vi "LOERN_AdaptToInputs.vi"(0 "XRef":T9, 1 "Term Types":T6, 2 "State In":T1={"Inputs"=1, "SelectedIndex"=0, "ClassInfo"=[]}) -> (14 "Reply":T4, 15 "Fatal Error Out":T3, 16 "State Out":T1={"Inputs"=1, "SelectedIndex"=0, "ClassInfo"=[]})   [LabVIEW 2016, in "LV Object Event Registration Node.xnode"]
uses:
  LV Object Event Registration Node.xnode
  <vilib>/XNodeSupport/XNodeXNodeRef.ctl
  <vilib>/XNodeSupport/XNodeTermTypeIDPairs.ctl
  <vilib>/XNodeSupport/XNodeTermTypeIDPair.ctl
  <vilib>/XNodeSupport/XNodeType.ctl
  <vilib>/XNodeSupport/XNodeString.ctl
  LOERN_State.ctl
  LOERN_ClassInfo.ctl
  <vilib>/XNodeSupport/XNodeStringArray.ctl
  <vilib>/XNodeSupport/XNodeErrorCluster.ctl
  <vilib>/Utility/Data Type/NI_Data Type.lvlib
  <vilib>/XNodeSupport/NI_XNodeSupport.lvlib
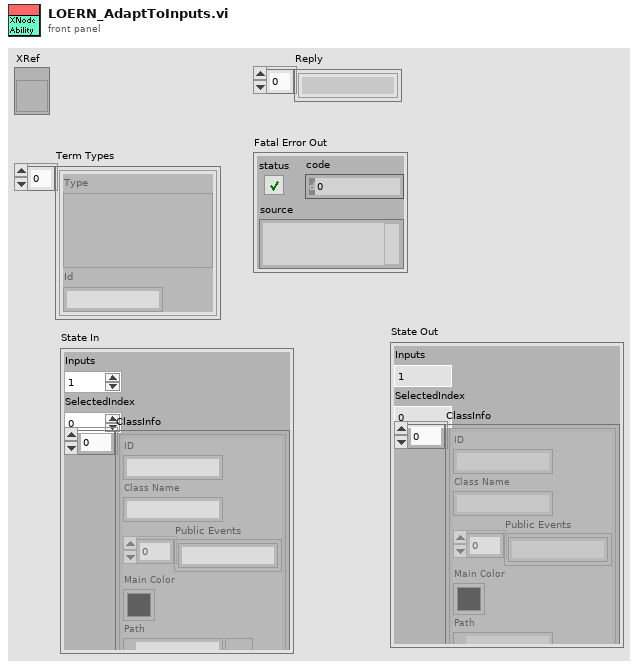
[diagram p1: front panel]
types:
  T1 = typedef "LV Object Event Registration Node.xnode/LOERN_State.ctl" = cluster{"Inputs":u16, "SelectedIndex":i16, "ClassInfo":T2[]}
  T2 = typedef "LV Object Event Registration Node.xnode/LOERN_ClassInfo.ctl" = cluster{"ID":string, "Class Name":string, "Public Events":string[], "Main Color":u32, "Path":path}
  T3 = typedef "NI_XNodeSupport.lvlib/XNodeErrorCluster.ctl" = errorcluster
  T4 = typedef "NI_XNodeSupport.lvlib/XNodeStringArray.ctl" = T5[]
  T5 = typedef "NI_XNodeSupport.lvlib/XNodeString.ctl" = string
  T6 = typedef "NI_XNodeSupport.lvlib/XNodeTermTypeIDPairs.ctl" = T7[]
  T7 = typedef "NI_XNodeSupport.lvlib/XNodeTermTypeIDPair.ctl" = cluster{"Type":T8, "Id":T5}
  T8 = typedef "NI_XNodeSupport.lvlib/XNodeType.ctl" = variant
  T9 = typedef "NI_XNodeSupport.lvlib/XNodeXNodeRef.ctl" = refnum<vi>
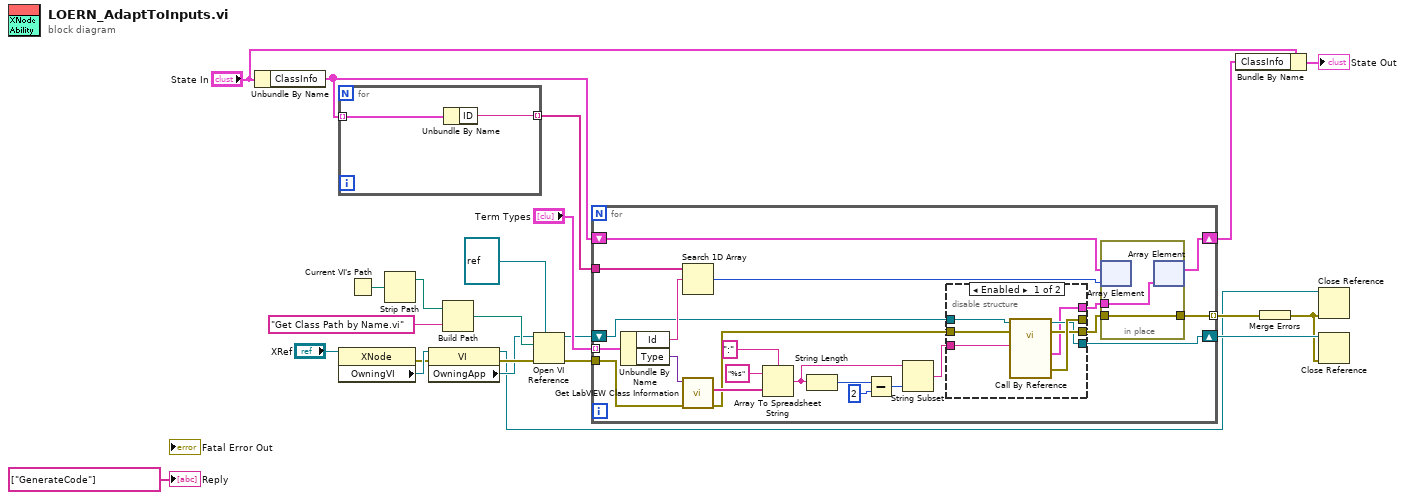
[diagram p0: block diagram]
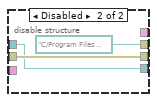
[diagram p2: hidden frame]
diagram:
  n1 = Unbundle By Name("State In") -> ("ClassInfo"=w21:T2[])
  n2 = for {
    tunnel: w21 -> [w25] mode=indexing
    tunnel: [w24] -> w22 mode=indexing
    n3 = Unbundle By Name(w25) -> ("ID"=w24:string)
  }
  n4 = property class="XNode"(reference="XRef") -> (error out=w12:errorcluster, "OwningVI"=w17:refnum<vi>)  [unwired: 1 in, 1 out]
  n5 = Current VI's Path() -> (path=w11:path)
  n6 = Strip Path(path=w11) -> (stripped path=w10:path)  [unwired: 1 out]
  n7 = property class="VI"(reference=w17, error in=w12) -> (reference out=w2:refnum<vi>, error out=w13:errorcluster, "OwningApp"=w7:refnum<vi>)
  n8 = Build Path(base path=w10, name or relative path="Get Class Path by Name.vi") -> (appended path=w8:path)
  n9 = Open VI Reference(type specifier VI Refnum (for type only)=refnum<vi> refnum, application reference (local)=w7, vi path=w8, error in (no error)=w13) -> (vi reference=w15:refnum<vi>, error out=w14:errorcluster)  [unwired: 2 in]
  n10 = for {
    tunnel: "Term Types" -> [w47] mode=indexing
    tunnel: w22 -> [w46]
    shift-right: [w42] -> w19
    shift-left: w21 -> [w44]
    tunnel: w14 -> [w29]
    shift-right: [w28] -> w5
    shift-left: w15 -> [w41]
    tunnel: [w27] -> w4 mode=indexing
    n11 = Unbundle By Name(w47) -> ("Id"=w45:T5, "Type"=w40:T8)
    n12 = Search 1D Array(1D array=w46, element=w45) -> (index of element=w43:i32)  [unwired: 1 in]
    n13 = call <vilib>:"Get LabVIEW Class Information.vi"("error in (no error)"=w29, "Variant"=w40) -> ("error out"=w30:errorcluster, "Qualified LabVIEW Class Name"=w37:string[])  [unwired: 7 in, 1 out]
    n14 = Array To Spreadsheet String(delimiter (Tab)=":", array=w37, 3:"%s" ("format string")) -> (spreadsheet string=w36:string)
    n15 = String Length(string=w36) -> (length=w35:i32)
    n16 = Subtract(x=w35, y=2) -> (x-y=w33:i32)
    n17 = String Subset(string=w36, length (rest)=w33) -> (substring=w32:string)  [unwired: 1 in]
    n18 = disable-structure shown="Enabled" {
      disable-tunnel: w41 -> [w54 w55]
      disable-tunnel: [w53 path "C:/Program Files (x86)/National Instruments/LabVIEW 2016/vi.lib/LIEF/Image Editor Handler/Image Editor Handler.lvclass"] -> _
      disable-tunnel: w32 -> [w52 _]
      disable-tunnel: [w51 w56] -> w31
      disable-tunnel: w30 -> [w50 w56]
      disable-tunnel: [w49 w55] -> w28
      disable-tunnel: [w48 _] -> w26
      frame Enabled {
        n19 = call-by-ref "?"(reference=w54, error in=w50, "String"=w52) -> (reference out=w49:refnum<vi>, error out=w51:errorcluster, "Error out"=w53:errorcluster, "output cluster"=w48:T2)  [unwired: 9 in]
      }
      frame Disabled {
      }
    }
    n20 = in-place {
      in-place-border: w31 -> [w59]
      in-place-border: [w59] -> w27
      in-place-border: w26 -> [w58]
      n21 = in-place-array #1(w44, w43) -> ()  [unwired: 1 out]
      n22 = in-place-array #1(w58) -> (w42:T2[])  [unwired: 1 out]
    }
  }
  n23 = Bundle By Name(cluster="State In", "ClassInfo"=w19) -> (→"State Out":T1)
  n24 = Merge Errors(w4) -> (w3:errorcluster)
  n25 = Close Reference(reference=w2, error in (no error)=w3) -> ()  [unwired: 1 out]
  n26 = Close Reference(reference=w5, error in (no error)=w3) -> ()  [unwired: 1 out]
  "Reply" <- T4 ["GenerateCode"] ("Reply")
